vi "tdms_testing.vi"() -> ()   [LabVIEW 2011]
panel:
  out "size(s)":i32
  in  "Array":T1(array[cluster])
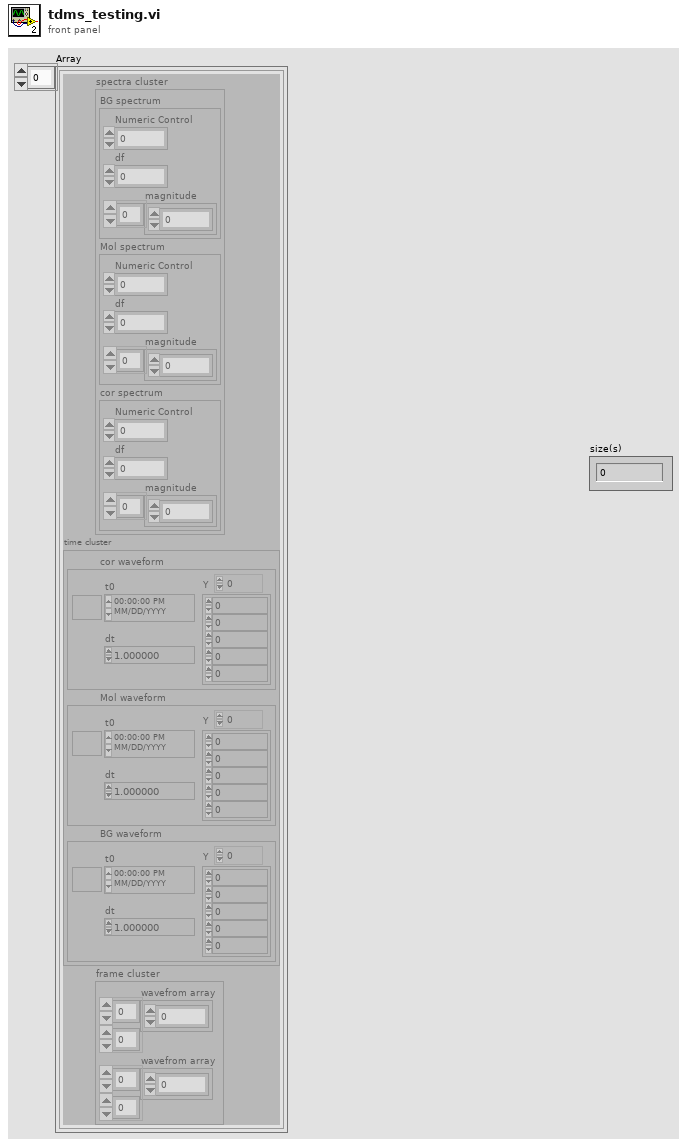
[diagram p1: front panel]
types:
  T1 = cluster{"spectra cluster":cluster{"BG spectrum":cluster{"Numeric Control":dbl, "df":dbl, "magnitude":dbl[]}, "Mol spectrum":cluster{"Numeric Control":dbl, "df":dbl, "magnitude":dbl[]}, "cor spectrum":cluster{"Numeric Control":dbl, "df":dbl, "magnitude":dbl[]}}, "time cluster":cluster{"cor waveform":waveform(dbl), "Mol waveform":waveform(dbl), "BG waveform":waveform(dbl)}, "frame cluster":cluster{"wavefrom array":dbl[][], "wavefrom array":dbl[][]}}[]
  T2 = enum16{"open", "open or create", "create or replace", "create", "open (read-only)"}
  T3 = cluster{"cor waveform":waveform(dbl), "Mol waveform":waveform(dbl), "BG waveform":waveform(dbl)}
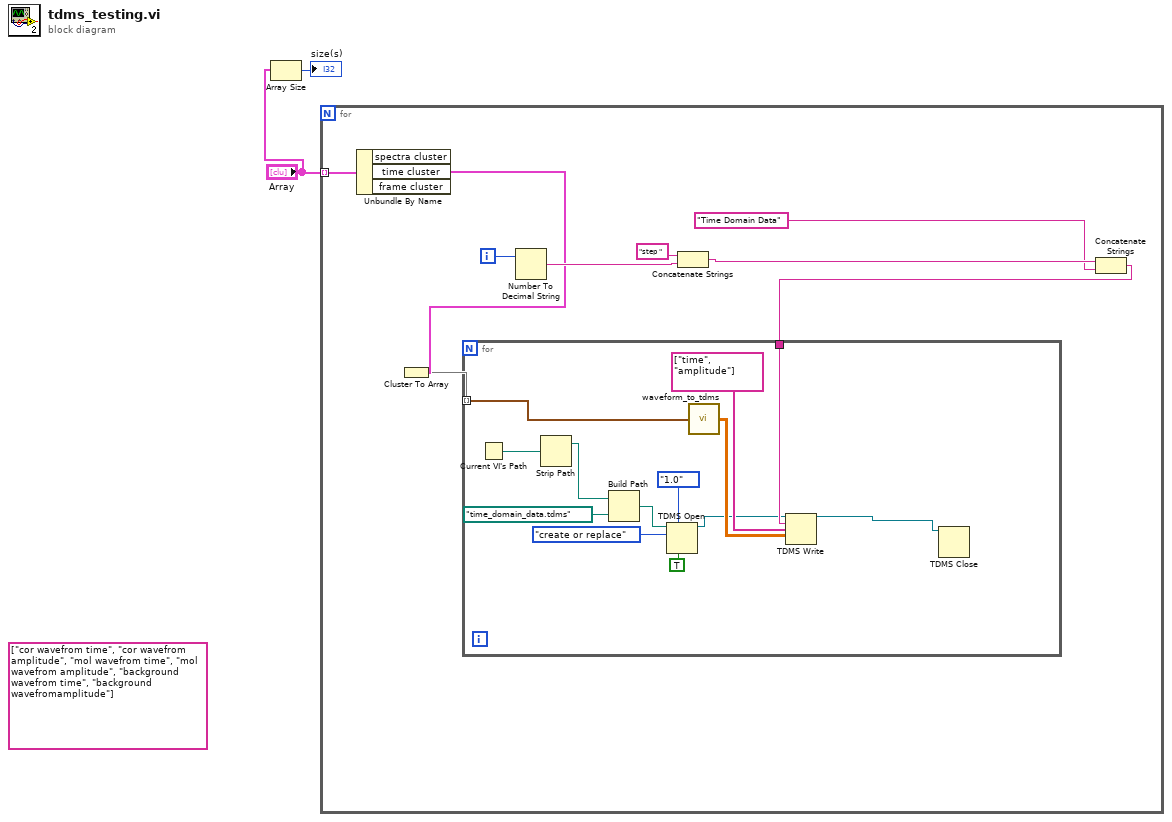
[diagram p0: block diagram]
diagram:
  (unwired) string[] ["cor wavefrom time", "cor wavefrom amplitude", "mol wavefrom time", "mol wavefrom amplitude", "background wavefrom time", "background wavefromamplitude"] ("channel name(s) in (Untitled)")
  n1 = Array Size(array="Array") -> (size(s)=→"size(s)":i32)
  n2 = for {
    tunnel: "Array" -> [w11] mode=indexing
    i -> [w10]
    n3 = Unbundle By Name(w11) -> ("time cluster"=w5:T3)  [unwired: 2 out]
    n4 = Cluster To Array(cluster=w5) -> (array=w4:waveform(dbl)[])
    n5 = Number To Decimal String(number=w10) -> (decimal integer string=w8:string)  [unwired: 1 in]
    n6 = Concatenate Strings("step " ("string"), w8) -> (w7:string)
    n7 = Concatenate Strings(w7, "Time Domain Data" ("group name in (Untitled)")) -> (w3:string)
    n8 = for {
      tunnel: w4 -> [w24] mode=indexing
      tunnel: w3 -> [w22]
      n9 = Current VI's Path() -> (path=w15:path)
      n10 = Strip Path(path=w15) -> (stripped path=w14:path)  [unwired: 1 out]
      n11 = Build Path(base path=w14, name or relative path=path "time_domain_data.tdms" ("file path")) -> (appended path=w18:path)
      n12 = TDMS Open(6:TRUE ("disable buffering (T)"), 7:enum16{"1.0", "2.0"}."1.0" ("file format version (2.0)"), 10:T2."create or replace" ("operation"), 11:w18) -> (3:w13:refnum<k34>)  [unwired: 2 in, 1 out]
      n13 = call "waveform_to_tdms.vi"("waveform"=w24) -> ("appended time data"=w23:dbl[][])  [unwired: 4 in]
      n14 = TDMS Write(0:w13, 5:w22, 7:string[] ["time", "amplitude"] ("channel name(s) in (Untitled)"), 9:w23) -> (4:w12:refnum<k34>)  [unwired: 2 in, 3 out]
      n15 = TDMS Close(11:w12) -> ()  [unwired: 1 in, 2 out]
    }
  }
